vi "write.vi"(8 "error in":errorcluster, 10 "element":T1, 11 "stream publisher in":refnum<class "subscriber.lvclass">) -> (0 "error out":errorcluster, 1 "timed out?":bool, 3 "stream publisher out":refnum<class "subscriber.lvclass">)   [LabVIEW 2013, in "data stream.lvlib" / "subscriber.lvclass"]
uses:
  subscriber.lvclass
  stream definition.ctl
  message definition.ctl
  subscriber.lvclass/subscriber.ctl
  data stream.lvlib
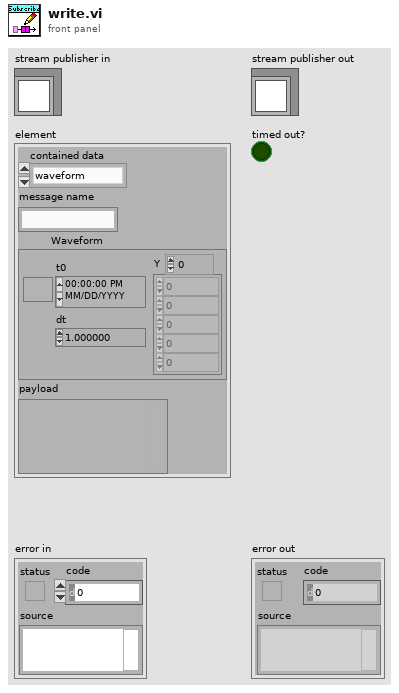
[diagram p1: front panel]
types:
  T1 = typedef "data stream.lvlib/stream definition.ctl" = cluster{"contained data":T2, "message name":string, "Waveform":waveform(dbl), "payload":variant}
  T2 = typedef "data stream.lvlib/message definition.ctl" = enum16{"waveform", "message"}
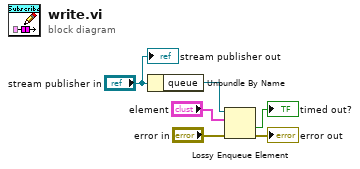
[diagram p0: block diagram]
diagram:
  n1 = Unbundle By Name("stream publisher in") -> ("queue"=w3:refnum<queue>)
  n2 = Lossy Enqueue Element(queue=w3, element="element", error in (no error)="error in") -> (overflow?=→"timed out?":bool, error out=→"error out":errorcluster)  [unwired: 2 out]
  "stream publisher out" <- "stream publisher in"
